vi "Bench_DURIP_Scheduling.vi"() -> ()   [LabVIEW 2023]
panel:
  out "output 1":timestamp=timestamp(3713988100 s since 1904-01-01)
  out "current time":timestamp=timestamp(3713988107.733025 s since 1904-01-01)
  out "x < y?":bool
  out "size(s)":i32[](array[numeric])=[3, 2]
  in  "Array":string[][](array[string])=[["24:21:40 9/8/2021", "temp1.bin"], ["22:59:41 9/8/2021", "temp45.bin"], ["22:59:42 9/8/2021", "temp45.bin"]]
  in  "stop":bool
  out "Time from string":timestamp=timestamp(3713986780 s since 1904-01-01)
  in  "String in HH:MM:SS.SSS MM/DD/YYYY Format":string="22:59:40 9/8/2021"
  # "Code detects when the transmission time is less than the clock but the transmission time + 1 second is greater\nthan the clock. When this condition is met, its time to transmit the file.\n\nTo Do 9/28/2021:\nCreate a subvi that will take a filename as input and transmit it, storing the resulting data. The subvi returns \nthe filename of the stored data and the time of the first data sample."
  # "Transmission Time"
  # "Transmission File"
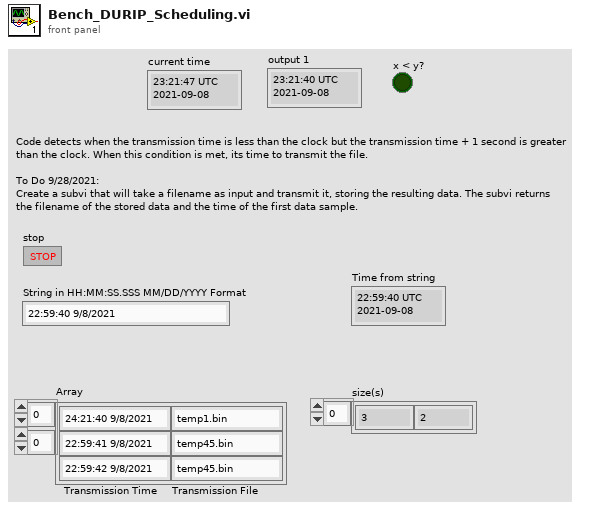
[diagram p1: front panel]
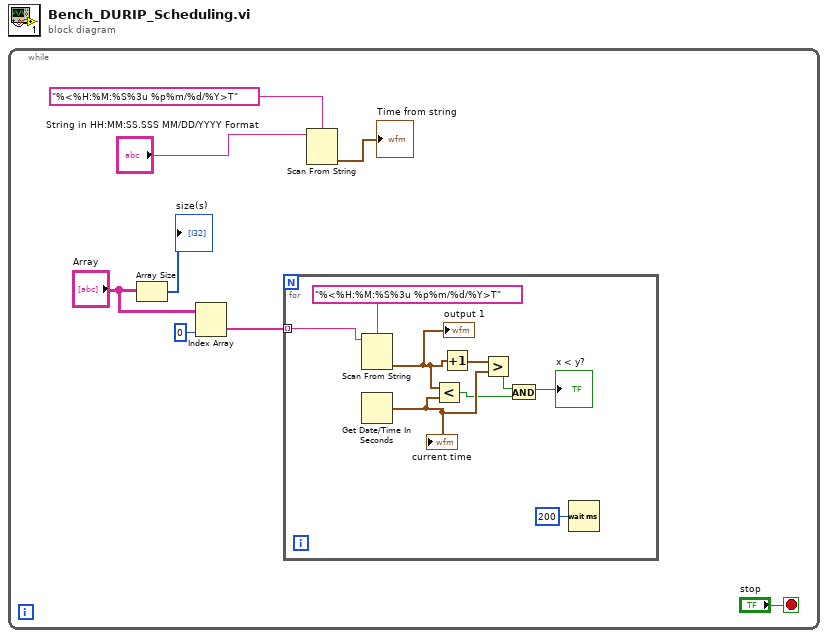
[diagram p0: block diagram]
diagram:
  n1 = while {
    stop <- "stop" stop-if-true
    n2 = Array Size(array="Array") -> (size(s)=→"size(s)":i32[])
    n3 = Index Array(array="Array", index (col)=0 ("disabled index (col)")) -> (element=w1:string[])  [unwired: 1 in]
    n4 = for {
      tunnel: w1 -> [w16] mode=indexing
      n5 = Scan From String(format string="%<%H:%M:%S%3u %p%m/%d/%Y>T", input string=w16) -> (output 1=w14:timestamp)  [unwired: 3 in, 3 out]
      "output 1" <- w14
      n6 = Get Date/Time In Seconds() -> (seconds since 1Jan1904=w12:timestamp)
      "current time" <- w12
      n7 = Less?(x=w14, y=w12) -> (x < y?=w10:bool)
      n8 = Increment(x=w14) -> (x+1=w13:timestamp)
      n9 = Greater?(x=w13, y=w12) -> (0:w11:bool)
      n10 = And(x=w11, y=w10) -> (x .and. y?=→"x < y?":bool)
      n11 = Wait (ms)(milliseconds to wait=u32 200) -> ()  [unwired: 1 out]
    }
    n12 = Scan From String(format string="%<%H:%M:%S%3u %p%m/%d/%Y>T", input string="String in HH:MM:SS.SSS MM/DD/YYYY Format") -> (output 1=→"Time from string":timestamp)  [unwired: 3 in, 3 out]
  }
